vi "Do.vi"(8 "error in (no error)":errorcluster, 10 "Actor in":refnum<class "Actor.lvclass">, 11 "Save to file Msg":refnum<class "Save to file Msg.lvclass">) -> (0 "error out":errorcluster, 2 "Actor out":refnum<class "Actor.lvclass">)   [LabVIEW 2020, in "Log.lvlib" / "Save to file Msg.lvclass"]
doc: "This VI delivers the message to the actor by calling the appropriate method(s) on the actor."
uses:
  Save to file Msg.lvclass
  <vilib>/ActorFramework/Actor/Actor.lvclass
  Save to file Msg.lvclass/Save to file Msg.ctl
  Log/Log.lvclass
  C:/Program Files (x86)/National Instruments/LabVIEW 2020/vi.lib/ActorFramework/Actor/Actor.lvclass
  9ef47adc-f318-494c-9b8b-6df3216d6863.vi
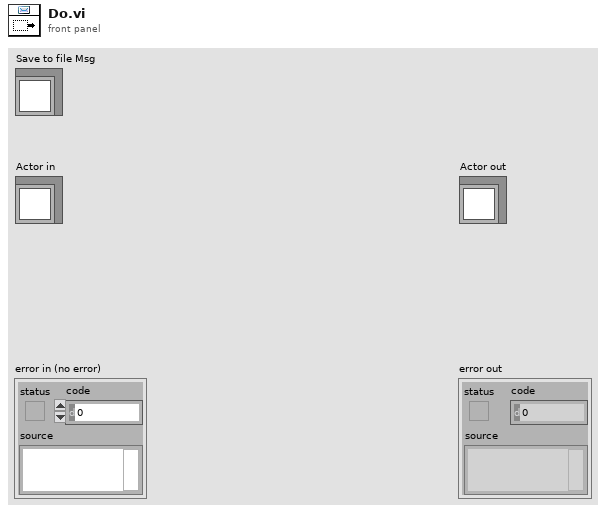
[diagram p1: front panel]
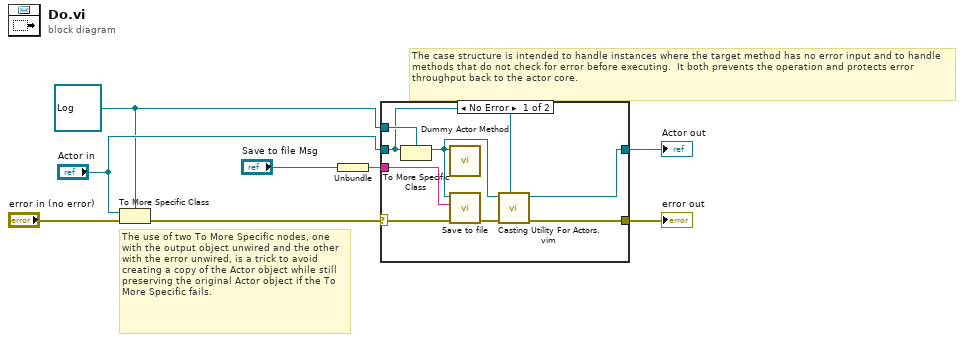
[diagram p0: block diagram]
diagram:
  w2 = refnum<class "Log.lvclass"> refnum ("Actor in")
  # "The use of two To More Specific nodes, one with the output object unwired and the other with the error unwired, is a trick to avoid creating a copy of the Actor object while still preserving the original Actor object if the To More Specific fails."
  # "The case structure is intended to handle instances where the target method has no error input and to handle methods that do not check for error before executing.  It both prevents the operation and protects error throughput back to the actor core."
  n1 = To More Specific Class(target class=w2, reference="Actor in", error in="error in (no error)") -> (error out=w6:errorcluster)  [unwired: 1 out]
  n2 = Unbundle("Save to file Msg") -> (w1:string)
  n3 = case shown="No Error" w6 {
    selector: w6 -> [w16 w18]
    tunnel: [w11 w18] -> w5
    tunnel: [w12 w17] -> w4
    tunnel: "Actor in" -> [w13 w17]
    tunnel: w2 -> [w14 _]
    tunnel: w1 -> [w9 _]
    frame No Error {
      n4 = To More Specific Class(target class=w14, reference=w13) -> (specific class reference=w15:refnum<class "Log.lvclass">)  [unwired: 1 in, 1 out]
      n5 = call <resource>:"Dummy Actor Method.vi"("Actor in"=w15) -> ()  [unwired: 9 in, 2 out]
      n6 = call "Save to file.vi"("error in (no error)"=w16, "Sent By"=w9, "Log in"=w15) -> ("error out"=w10:errorcluster)  [unwired: 8 in]
      n7 = call "Casting Utility For Actors.vim"("type"=w13, "error in (no error)"=w10, "Actor in"=w15) -> ("error out"=w11:errorcluster, "Actor out"=w12:refnum<class "Actor.lvclass">)  [unwired: 7 in]
    }
    frame Error {
      # "If type check fails, pass the original object out again."
    }
  }
  "error out" <- w5
  "Actor out" <- w4
